vi "Read Speed [km_h].vi"(8 "error in (no error)":errorcluster, 11 "Spaceship in":refnum<class "Spaceship.lvclass">) -> (0 "error out":errorcluster, 2 "Speed [km/h]":dbl, 3 "Spaceship out":refnum<class "Spaceship.lvclass">)   [LabVIEW 2021, in "Spaceship.lvclass"]
uses:
  Spaceship.lvclass
  Spaceship.lvclass/Spaceship.ctl
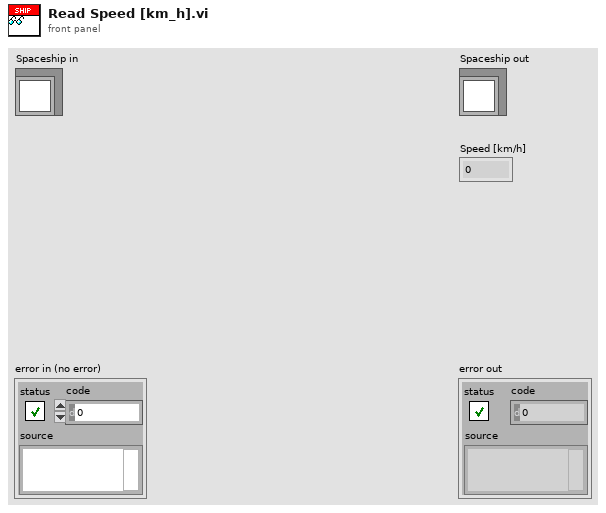
[diagram p1: front panel]
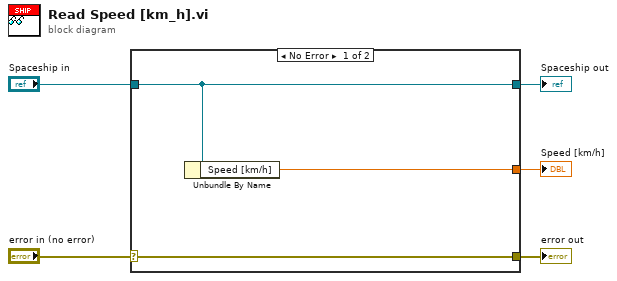
[diagram p0: block diagram]
diagram:
  n1 = case shown="No Error" "error in (no error)" {
    selector: "error in (no error)" -> [w8 w9]
    tunnel: [w8 w9] -> w4
    tunnel: [w7 w10] -> w2
    tunnel: "Spaceship in" -> [w7 w10]
    tunnel: [w6 _] -> w1
    frame No Error {
      n2 = Unbundle By Name(w7) -> ("Speed [km/h]"=w6:dbl)
    }
    frame Error {
    }
  }
  "error out" <- w4
  "Spaceship out" <- w2
  "Speed [km/h]" <- w1
